vi "BlackBodyFurnace Visualization.vi"() -> ()   [LabVIEW 2018]
uses:
  <resource>/objmgr/daqmx.rc
panel:
  out "element":cluster{dbl[], dbl[]}
  out "XY Graph 3":cluster{dbl[], dbl[]}(graph)
  out "XY Graph 2":cluster{dbl[], dbl[]}(graph)
  in  "Reset":bool=TRUE
  out "XY Graph":cluster{"Y":dbl[], "Y":dbl[]}[](graph)
  in  "stop":bool
  in  "DAQmx Task Name":refnum<k21>="TC1"
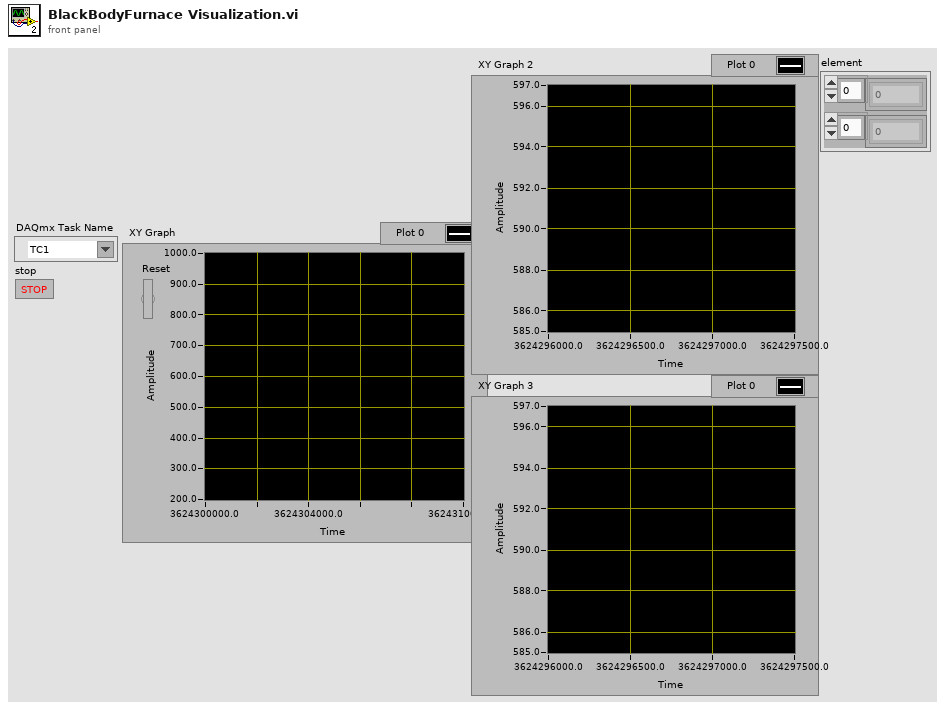
[diagram p1: front panel]
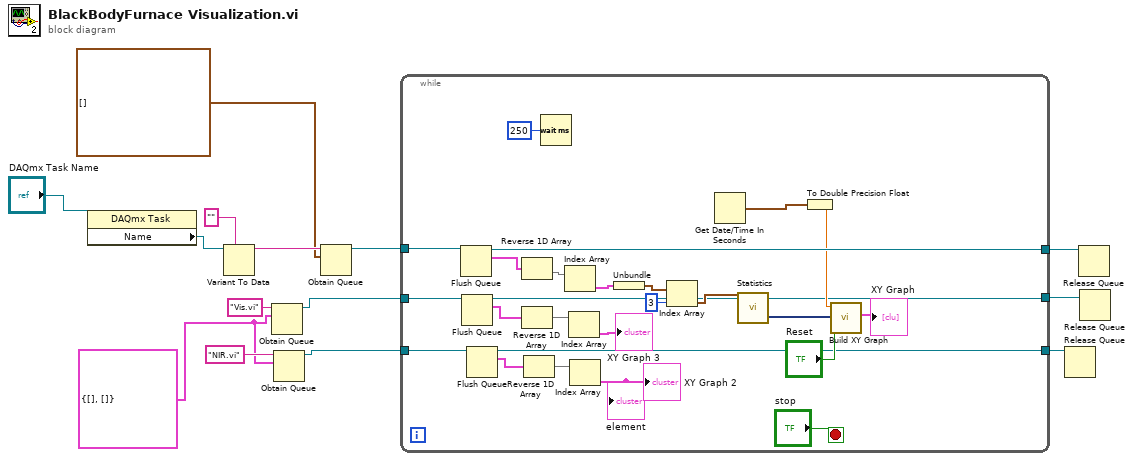
[diagram p0: block diagram]
diagram:
  w1 = cluster{dbl[], dbl[]} {[], []}
  n1 = property class="DAQmx Task"(reference="DAQmx Task Name") -> ("Name"=w13:refnum<k21>)  [unwired: 1 in, 2 out]
  n2 = Variant To Data(type="", Variant=w13) -> (data=w11:string)  [unwired: 1 in, 1 out]
  n3 = Obtain Queue(name (unnamed)="Vis.vi", element data type=w1) -> (queue out=w5:refnum<queue>)  [unwired: 3 in, 2 out]
  n4 = Obtain Queue(name (unnamed)="NIR.vi", element data type=w1) -> (queue out=w4:refnum<queue>)  [unwired: 3 in, 2 out]
  n5 = Obtain Queue(name (unnamed)=w11, element data type=waveform(dbl)[] [] ("data")) -> (queue out=w9:refnum<queue>)  [unwired: 3 in, 2 out]
  n6 = while {
    tunnel: w9 -> [w39]
    tunnel: [w33] -> w8
    tunnel: w5 -> [w24]
    tunnel: w4 -> [w23]
    tunnel: [w18] -> w3
    tunnel: [w17] -> w2
    stop <- "stop" stop-if-true
    n7 = Flush Queue(queue=w39) -> (queue out=w33:refnum<queue>, remaining elements=w38:cluster{"data":waveform(dbl)[]}[])  [unwired: 1 in, 1 out]
    n8 = Flush Queue(queue=w24) -> (queue out=w18:refnum<queue>, remaining elements=w21:cluster{dbl[], dbl[]}[])  [unwired: 1 in, 1 out]
    n9 = Flush Queue(queue=w23) -> (queue out=w17:refnum<queue>, remaining elements=w22:cluster{dbl[], dbl[]}[])  [unwired: 1 in, 1 out]
    n10 = Reverse 1D Array(array=w38) -> (reversed array=w37:cluster{"data":waveform(dbl)[]}[])
    n11 = Reverse 1D Array(array=w21) -> (reversed array=w19:cluster{dbl[], dbl[]}[])
    n12 = Reverse 1D Array(array=w22) -> (reversed array=w20:cluster{dbl[], dbl[]}[])
    n13 = Wait (ms)(milliseconds to wait=u32 250) -> ()  [unwired: 1 out]
    n14 = Index Array(array=w37) -> (element=w36:cluster{"data":waveform(dbl)[]})  [unwired: 1 in]
    n15 = Index Array(array=w19) -> (element=→"XY Graph 3":cluster{dbl[], dbl[]})  [unwired: 1 in]
    n16 = Index Array(array=w20) -> (element=→"XY Graph 2" →"element":cluster{dbl[], dbl[]})  [unwired: 1 in]
    n17 = Unbundle(w36) -> ("data"=w35:waveform(dbl)[])
    n18 = Index Array(array=w35, index=3) -> (element=w30:waveform(dbl))
    n19 = Get Date/Time In Seconds() -> (seconds since 1Jan1904=w27:timestamp)
    n20 = call "Statistics"("Signals"=w30) -> ("Arithmetic Mean"=w28:dynamicdata)  [unwired: 25 in, 1 out]
    n21 = To Double Precision Float(number=w27) -> (double precision float=w26:dbl)
    n22 = call "Build XY Graph"("Reset"="Reset", "Y Input"=w28, "X Input"=w26) -> ("XY Graph"=→"XY Graph":cluster{"X":dbl[], "Y":dbl[]}[])  [unwired: 7 in, 1 out]
  }
  n23 = Release Queue(queue=w2) -> ()  [unwired: 2 in, 3 out]
  n24 = Release Queue(queue=w8) -> ()  [unwired: 2 in, 3 out]
  n25 = Release Queue(queue=w3) -> ()  [unwired: 2 in, 3 out]
